vi "TharOff.vi"(8 "Error In":errorcluster, 11 "Handle In":u32) -> (0 "Error Out":errorcluster, 3 "Handle Out":u32)   [LabVIEW 2016]
panel:
  out "concatenated string":string
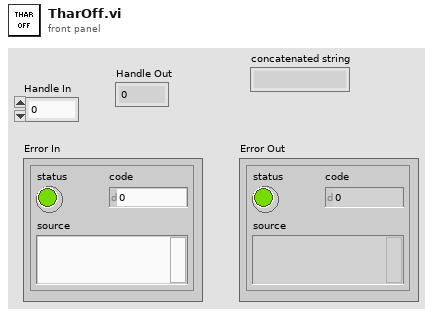
[diagram p1: front panel]
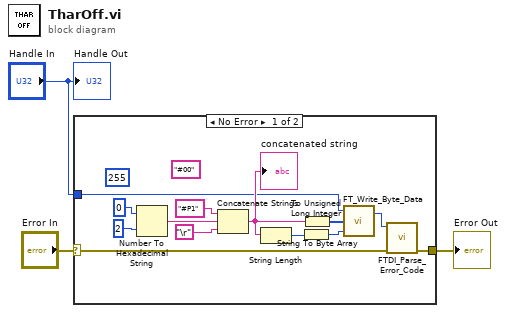
[diagram p0: block diagram]
diagram:
  n1 = case shown="No Error" "Error In" {
    selector: "Error In" -> [w5 w17]
    tunnel: "Handle In" -> [w9 _]
    tunnel: [w4 w17] -> w1
    frame No Error {
      (unwired) 255 ("number")
      (unwired) "#00" ("Substring")
      n2 = Number To Hexadecimal String(1:i16 2 ("width (-)"), 2:0 ("number")) -> (0:w15:string)
      n3 = Concatenate Strings("#P1" ("Substring"), w15, "\r") -> (w10:string)
      "concatenated string" <- w10
      n4 = String Length(string=w10) -> (length=w13:i32)
      n5 = To Unsigned Long Integer(number=w13) -> (unsigned 32bit integer=w12:u32)
      n6 = String To Byte Array(string=w10) -> (unsigned byte array=w11:u8[])
      n7 = call "FT_Write_Byte_Data.vi"("Bytes To Write"=w12, "Buffer"=w11, "Handle"=w9) -> ("FT_Status"=w6:u32)  [unwired: 1 out]
      n8 = call "FTDI_Parse_Error_Code.vi"("error in (no error)"=w5, "FT_Status"=w6) -> ("error out"=w4:errorcluster)  [unwired: 9 in]
    }
    frame Error {
    }
  }
  "Error Out" <- w1
  "Handle Out" <- "Handle In"
